vi "Start New File.vi"(8 "error in (no error)":errorcluster, 11 "Logger in":refnum<class "Logger.lvclass">) -> (0 "error out":errorcluster, 2 "File Path":path, 3 "Logger out":refnum<class "Logger.lvclass">)   [LabVIEW 2016, in "Logger.lvclass"]
uses:
  Logger.lvclass
  Logger.lvclass/Logger.ctl
  Read File.lvclass.vi
  Write File.lvclass.vi
  Write Last clean-up time stamp.vi
  NHMFL_Core/Libraries/File/File Class/File.lvclass
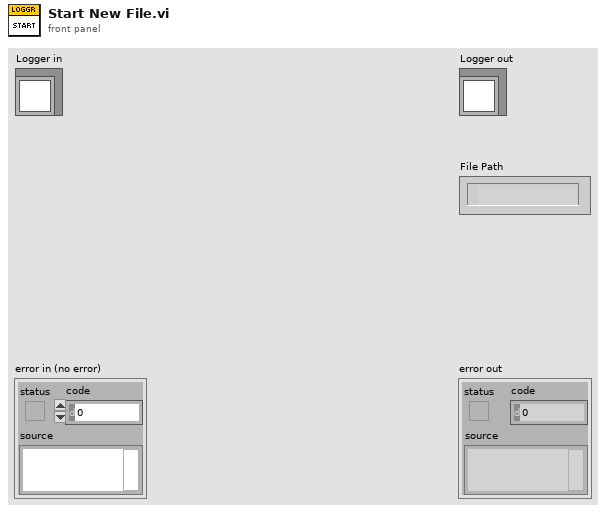
[diagram p1: front panel]
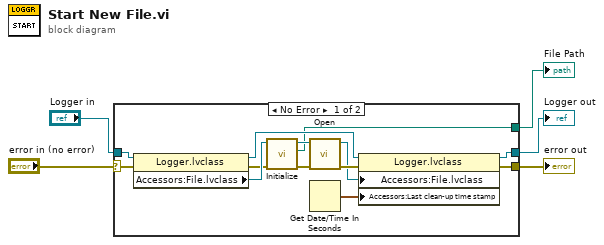
[diagram p0: block diagram]
diagram:
  n1 = case shown="No Error" "error in (no error)" {
    selector: "error in (no error)" -> [w18 w20]
    tunnel: [w13 w20] -> w4
    tunnel: [w12 w19] -> w2
    tunnel: "Logger in" -> [w17 w19]
    tunnel: [w7 _] -> w1
    frame No Error {
      n2 = property class="Logger.lvclass"(reference=w17, error in=w18) -> (reference out=w15:refnum<class "Logger.lvclass">, error out=w14:errorcluster, "Accessors:File.lvclass"=w16:refnum<class "File.lvclass">)
      n3 = call-dynamic "Initialize.vi"("error in (no error)"=w14, "File in"=w16) -> ("error out"=w10:errorcluster, "File Path"=w7:path, "File out"=w11:refnum<class "File.lvclass">)  [unwired: 7 in]
      n4 = call-dynamic "Open.vi"("error in (no error)"=w10, "File in"=w11) -> ("error out"=w9:errorcluster, "File out"=w8:refnum<class "File.lvclass">)  [unwired: 8 in]
      n5 = Get Date/Time In Seconds() -> (seconds since 1Jan1904=w6:timestamp)
      n6 = property class="Logger.lvclass"(reference=w15, error in=w9, "Accessors:File.lvclass"=w8, "Accessors:Last clean-up time stamp"=w6) -> (reference out=w12:refnum<class "Logger.lvclass">, error out=w13:errorcluster)
    }
    frame Error {
    }
  }
  "error out" <- w4
  "Logger out" <- w2
  "File Path" <- w1
